vi "Configure Pulse Width.vi"(4 "pulse number":i32=1 min=1 max=4, 6 "channel":i32=1 min=1 max=4, 8 "error in (no error)":errorcluster, 10 "pulse width (s)":dbl=0.005 min=0.005 max=5.0, 11 "VISA resource name":refnum<visa-resource-name>) -> (0 "error out":errorcluster, 3 "VISA resource name out":refnum<visa-resource-name>)   [LabVIEW 2019, in "Pulse Rider PG-1000.lvlib"]
doc: "Sets the pulse width for the specified pulse relative to the selected output channel.\n\nPulse Width = Period × Duty Cycle / 100. The pulse width must be less than the period. Pulse Width <= Pulse Period\n\nw: the pulse width in second\nchannel: the output channel int from 1 to 4\npulse_nb: the pulse number int from 1 to 4"
uses:
  <instrlib>/LV_PulseRiderPG1000/Pulse Rider PG-1000.lvlib
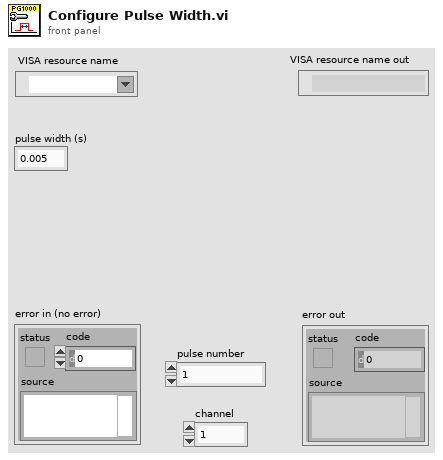
[diagram p1: front panel]
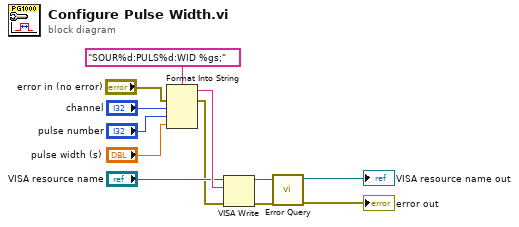
[diagram p0: block diagram]
diagram:
  n1 = Format Into String(format string="SOUR%d:PULS%d:WID %gs;", error in="error in (no error)", "channel", "pulse number", "pulse width (s)") -> (resulting string=w9:string, error out=w2:errorcluster)  [unwired: 1 in]
  n2 = VISA Write(VISA resource name="VISA resource name", write buffer=w9, error in (no error)=w2) -> (VISA resource name out=w12:refnum<visa-resource-name>, error out=w11:errorcluster)  [unwired: 1 out]
  n3 = call <instrlib>:"Error Query.vi"("error in (no error)"=w11, "VISA resource name"=w12) -> ("error out"=→"error out":errorcluster, "VISA resource name out"=→"VISA resource name out":refnum<visa-resource-name>)  [unwired: 6 in, 2 out]
